vi "Collision_get.vi"(8 "error in (no error)":errorcluster) -> (0 "error out":errorcluster, 2 "Collision":bool)   [LabVIEW 2009, in "NetworkVarTarget.lvlib"]
uses:
  NetworkVarTarget.lvlib
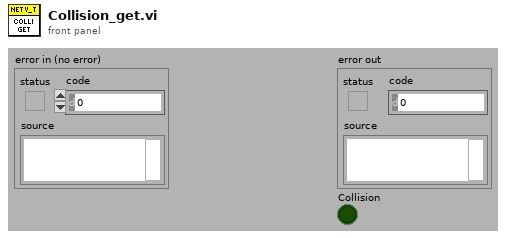
[diagram p1: front panel]
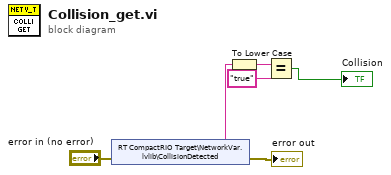
[diagram p0: block diagram]
diagram:
  n1 = shared-variable "RT CompactRIO Target\\NetworkVar.lvlib\\CollisionDetected"(error in="error in (no error)") -> (w4:string, error out=→"error out":errorcluster)
  n2 = To Lower Case(string=w4) -> (all lower case string=w3:string)
  n3 = Equal?(x=w3, y="true") -> (x = y?=→"Collision":bool)
